vi "CheesyDrive.vi"(4 "SlowRate?":bool, 5 "Quickturn":bool, 6 "Slowrate %0 - 100":dbl=60.0, 7 "WheelNonLinearity":dbl=0.75, 8 "negInertiaScalar":dbl=1.0, 9 "Sensitivty":dbl=1.1, 10 "Wheel":dbl(slide)=-0.08661417322834646 scale=-1.0..1.0, 11 "Throttle":dbl(slide)=0.031496062992125984 scale=-1.0..1.0) -> (2 "Right PWM":dbl, 3 "Left PWM":dbl)   [LabVIEW 2020]
doc: "Implements CheesyDrive. CheesyDrive means that the turn joystick controls the radius of turning instead of the rate of turning. Also implements QuickStop and QuickTurn."
panel:
  in  "Deadband 2":dbl=0.1 format="%#_13g"
  in  "Deadband":dbl=0.1 format="%#_13g"
  out "Right":dbl(slide) scale=-1.0..1.0
  out "Left":dbl(slide) scale=-1.0..1.0
  in  "CarLikeTurning":bool
  in  "QSMult":dbl=2.0
  in  "Max dx/dt":dbl=2.5
  in  "alpha":dbl=0.1
  out "r - out":dbl(graph)
  # "Enable to enable"
  # "(for quickstop decay)"
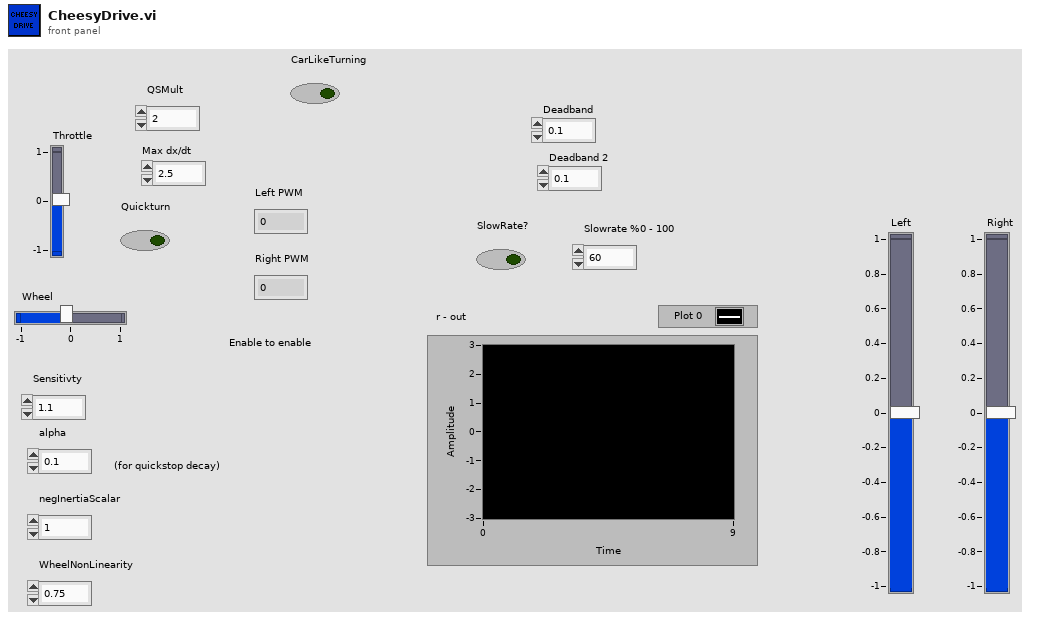
[diagram p1: front panel]
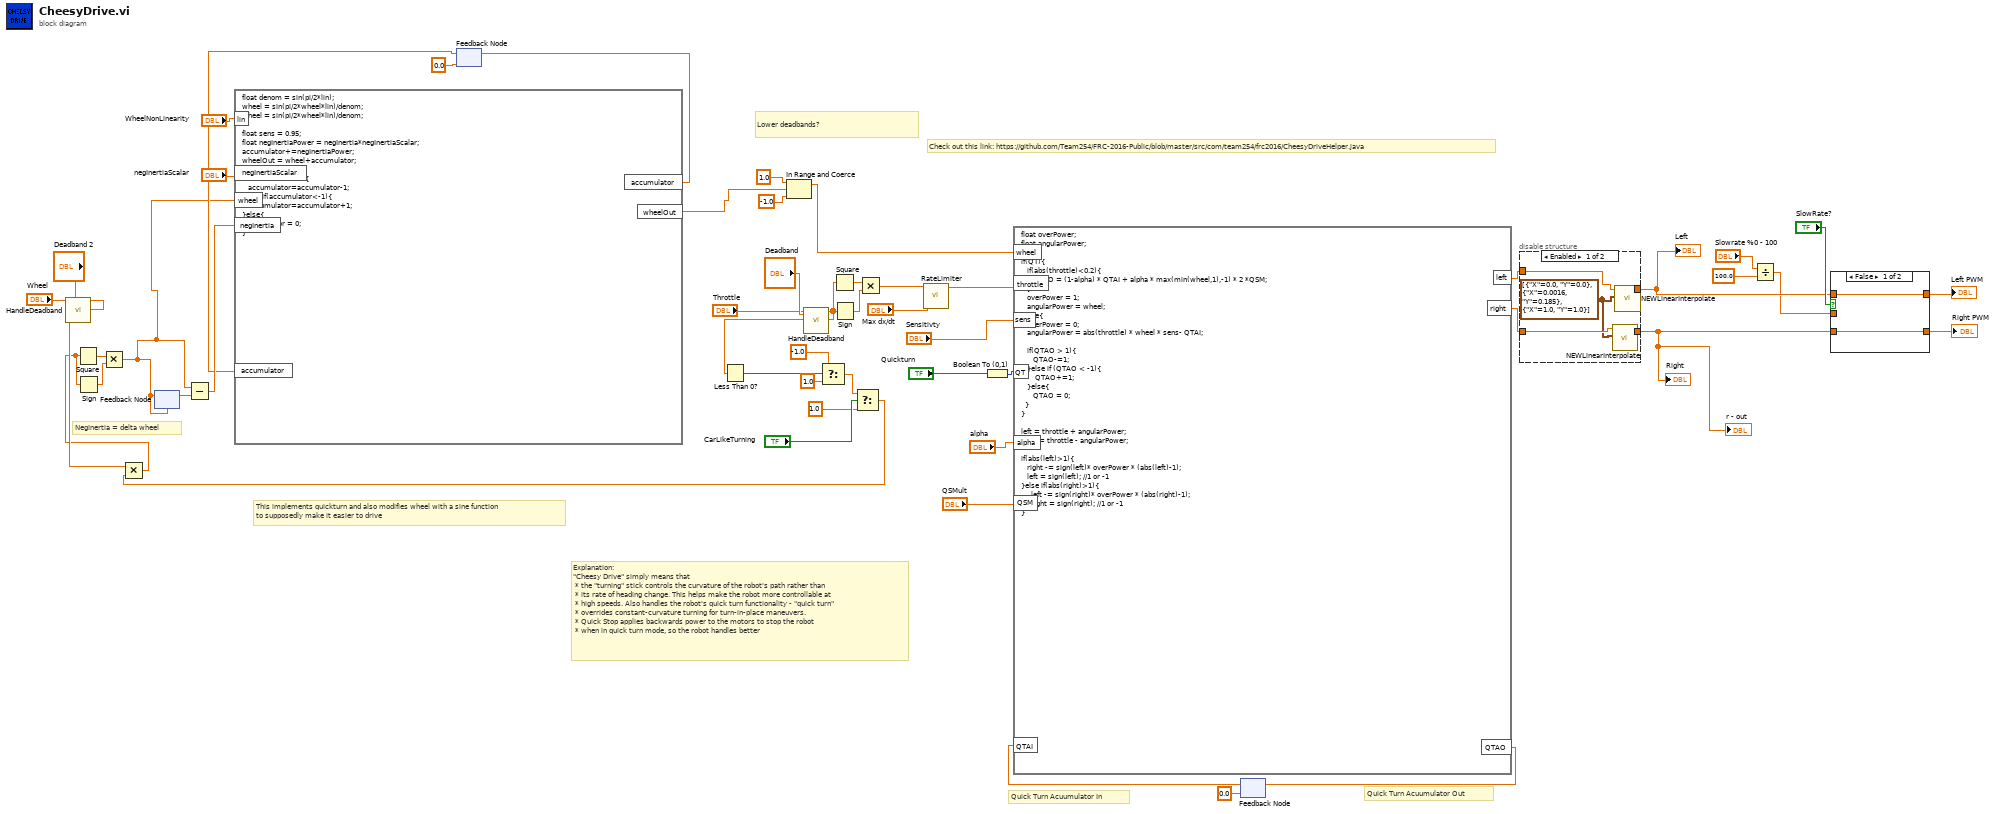
[diagram p0: block diagram]
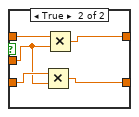
[diagram p2: hidden frame]
diagram:
  # "This implements quickturn and also modifies wheel with a sine function\nto supposedly make it easier to drive"
  # "Lower deadbands?"
  # "NegInertia = delta wheel"
  # "Explanation:\n\"Cheesy Drive\" simply means that\n * the \"turning\" stick controls the curvature of the robot's path rather than\n * its rate of heading change. This helps make the robot more controllable at\n * high speeds. Also handles the robot's quick turn functionality - \"quick turn\"\n * overrides constant-curvature turning for turn-in-place maneuvers.\n * Quick Stop applies backwards power to the motors to stop the robot\n * when in quick turn mode, so the robot handles better"
  # "Quick Turn Acuumulator Out"
  # "Quick Turn Acuumulator In"
  # "Check out this link: https://github.com/Team254/FRC-2016-Public/blob/master/src/com/team254/frc2016/CheesyDriveHelper.java"
  n1 = call "HandleDeadband.vi"("Deadband"="Deadband 2", "Input"="Wheel") -> ("Output"=w15:dbl)  [unwired: 9 in]
  n2 = feedback #1(0.0 ("Wheel")) -> (w33:dbl)
  n3 = call "HandleDeadband.vi"("Deadband"="Deadband", "Input"="Throttle") -> ("Output"=w16:dbl)  [unwired: 9 in]
  n4 = Less Than 0?(x=w16) -> (x < 0?=w19:bool)
  n5 = Select(t=-1.0, s=w19, f=1.0) -> (s? t:f=w11:dbl)
  n6 = Square(x=w16) -> (x^2=w42:dbl)
  n7 = Sign(1:w16) -> (0:w41:dbl)
  n8 = Select(t=w11, s="CarLikeTurning", f=1.0) -> (s? t:f=w9:dbl)
  n9 = Multiply(x=w15, y=w9) -> (x*y=w14:dbl)
  n10 = Square(x=w14) -> (x^2=w24:dbl)
  n11 = Sign(1:w14) -> (0:w23:dbl)
  n12 = Multiply(x=w24, y=w23) -> (x*y=w13:dbl)
  n13 = feedback #2(w13) -> (w35:dbl)
  n14 = feedback-in #2(w13) -> ()
  n15 = Subtract(x=w13, y=w35) -> (x-y=w34:dbl)
  n16 = formula code="float denom = sin(pi/2*lin);\nwheel = sin(pi/2*wheel*lin)/denom;\nwheel = sin(pi/2*wheel*lin)/denom;\n\nfloat sens = 0.95;\nfloat negInertiaPower = negInertia*negInertiaScalar;\naccumulator+=negInertiaPower;\nwheelOut = wheel+accumulator;\n\nif(accumulator>1){\n   accumulator=accumulator-1;\n}else if(accumulator<-1){\n   accumulator=accumulator+1;\n}else{\naccumulator = 0;\n}"("wheel"=w13, "negInertia"=w34, "accumulator"=w33, "negInertiaScalar"="negInertiaScalar", "lin"="WheelNonLinearity") -> ("accumulator"=w31:dbl, "wheelOut"=w25:dbl)
  n17 = feedback-in #1(w31) -> ()
  n18 = In Range and Coerce(upper limit=1.0, x=w25, lower limit=-1.0) -> (coerced(x)=w26:dbl)  [unwired: 1 out]
  n19 = Multiply(x=w42, y=w41) -> (x*y=w40:dbl)
  n20 = call "RateLimiter.vi"("Max dx/dt"="Max dx/dt", "Input"=w40) -> ("Output"=w39:dbl)  [unwired: 9 in]
  n21 = Boolean To (0,1)(Boolean="Quickturn") -> (0, 1=w46:i16)
  n22 = feedback #3(0.0 ("QTAccumulatorO")) -> (w44:dbl)
  n23 = formula code="float overPower;\nfloat angularPower;\n\nif(QT){\n   if(abs(throttle)<0.2){\n      QTAO = (1-alpha) * QTAI + alpha * max(min(wheel,1),-1) * 2 *QSM;\n   }\n   overPower = 1;\n   angularPower = wheel;\n}else{\n   overPower = 0;\n   angularPower = abs(throttle) * wheel * sens- QTAI;\n\n   if(QTAO > 1){\n      QTAO-=1;\n   }else if (QTAO < -1){\n       QTAO+=1;\n   }else{\n      QTAO = 0;\n  }\n}\n\nleft = throttle + angularPower;\nright = throttle - angularPower;\n\nif(abs(left)>1){\n   right -= sign(left)* overPower * (abs(left)-1);\n   left = sign(left); //1 or -1\n}else if(abs(right)>1){\n     left -= sign(right)* overPower * (abs(right)-1);\n     right = sign(right); //1 or -1 \n}"("wheel"=w26, "throttle"=w39, "sens"="Sensitivty", "QT"=w46, "alpha"="alpha", "QTAI"=w44, "QSM"="QSMult") -> ("left"=w37:dbl, "right"=w36:dbl, "QTAO"=w47:dbl)
  n24 = feedback-in #3(w47) -> ()
  n25 = disable-structure shown="Enabled" {
    disable-tunnel: w37 -> [w56 w58]
    disable-tunnel: [w55 w58] -> w7
    disable-tunnel: [w54 w57] -> w5
    disable-tunnel: w36 -> [w53 w57]
    frame Enabled {
      w52 = cluster{"X":dbl, "Y":dbl}[] [{"X"=0.0, "Y"=0.0}, {"X"=0.0016, "Y"=0.185}, {"X"=1.0, "Y"=1.0}] ("Points")
      n26 = call "NEWLinearInterpolate.vi"("Points"=w52, "Value"=w53) -> ("Output"=w54:dbl)  [unwired: 9 in]
      n27 = call "NEWLinearInterpolate.vi"("Points"=w52, "Value"=w56) -> ("Output"=w55:dbl)  [unwired: 9 in]
    }
    frame Disabled {
    }
  }
  "r - out" <- w5
  "Right" <- w5
  "Left" <- w7
  n28 = Divide(x="Slowrate %0 - 100", y=100.0) -> (x/y=w1:dbl)
  n29 = case shown="False" "SlowRate?" {
    tunnel: w7 -> [w60 w65]
    tunnel: [w60 w61] -> w6
    tunnel: w5 -> [w59 w64]
    tunnel: [w59 w62] -> w4
    tunnel: w1 -> [_ w63]
    frame False {
    }
    frame True {
      n30 = Multiply(x=w64, y=w63) -> (x*y=w62:dbl)
      n31 = Multiply(x=w65, y=w63) -> (x*y=w61:dbl)
    }
  }
  "Left PWM" <- w6
  "Right PWM" <- w4
